vi "Main.vi"() -> ()   [LabVIEW 2020, in "DQMH_API.lvlib"]
uses:
  DQMH_API.lvlib
  Event types--enum.ctl
panel:
  in  "Events":u16(ring) items=["Cloneable Module.lvlib:Do Something.vi", "Cloneable Module.lvlib:Do Something Else.vi", "Cloneable Module.lvlib:Show Panel.vi", "Cloneable Module.lvlib:Hide Panel.vi", "Cloneable Module.lvlib:Stop Module.vi", "Cloneable Module.lvlib:Show Diagram.vi"]
  in  "Event type":T1
  in  "Scan Module Events":bool
  in  "Stop":bool
  in  "Module to work with":u16(ring) items=["Singleton Module.lvlib", "Cloneable Module.lvlib"]
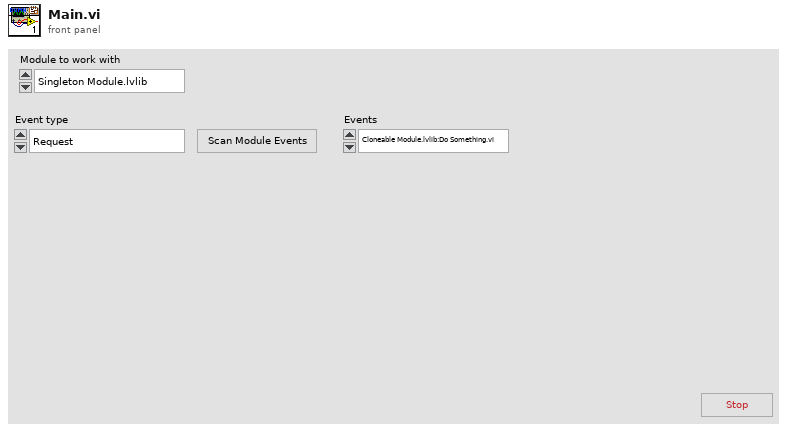
[diagram p1: front panel]
types:
  T1 = typedef "DQMH_API.lvlib/Event types--enum.ctl" = enum16{"Request", "Request and Wait for Reply", "Broadcast"}
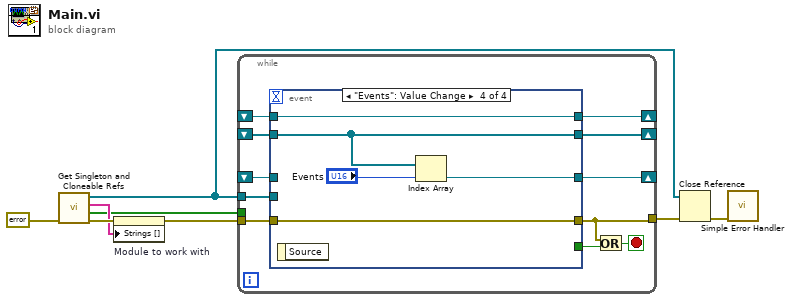
[diagram p0: block diagram]
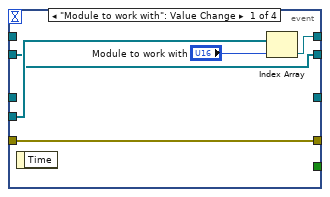
[diagram p2: hidden frame]
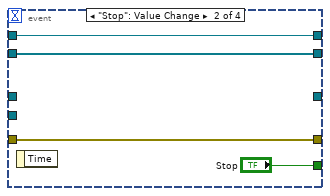
[diagram p3: hidden frame]
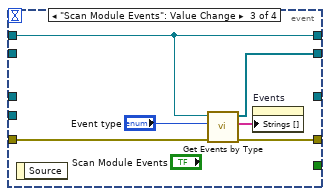
[diagram p4: hidden frame]
diagram:
  n1 = call "Get Singleton and Cloneable Refs.vi"("error in"=errorcluster {"status"=FALSE, "code"=0, "source"=""}) -> ("error out"=w6:errorcluster, "Cloneable?"=w2:bool[], "Modules List"=w3:string[], "DQMH Modules"=w1:refnum<vi>[])  [unwired: 7 in]
  n2 = property on="Module to work with" class="Ring (strict)"(error in=w6, "Strings []"=w3) -> (error out=w7:errorcluster)  [unwired: 1 in, 1 out]
  n3 = while {
    tunnel: w1 -> [w17]
    tunnel: w7 -> [w19]
    tunnel: w2 -> [_]
    tunnel: [w18] -> w5
    shift-right: [w15] -> _
    shift-left: _ -> [w13]
    shift-right: [w12] -> _
    shift-left: _ -> [w11]
    shift-right: [w10] -> _
    shift-left: _ -> [w9]
    stop <- w14 stop-if-true
    n4 = event shown="[3] \"Events\": Value Change" {
      selector: _ -> [_ _ _ _]
      dyn-events: _ -> [_ _ _ _]
      timeout: _ -> [_ _ _ _]
      tunnel: w17 -> [w23 _ _ _]
      tunnel: [_ "Stop" _ _] -> w16
      tunnel: [w21 w26 w31 w37] -> w15
      tunnel: w19 -> [w24 w28 w34 w36]
      tunnel: [w24 w28 w33 w36] -> w18
      tunnel: w13 -> [_ w26 w31 w37]
      tunnel: [w20 w25 w29 w38] -> w12
      tunnel: w11 -> [w20 w25 _ w38]
      tunnel: [_ _ _ w35] -> w10
      tunnel: w9 -> [_ _ _ _]
      event "Module to work with": Value Change {
        n5 = event-data() -> ()  [unwired: 1 in, 1 out]
        n6 = Index Array(array=w23, index="Module to work with") -> (element=w21:refnum<vi>)
      }
      event "Stop": Value Change {
        n7 = event-data() -> ()  [unwired: 1 in, 1 out]
      }
      event "Scan Module Events": Value Change {
        n8 = event-data() -> ()  [unwired: 1 in, 1 out]
        n9 = call "Get Events by Type.vi"("error in"=w34, "Event type"="Event type", "DQMH Module Ref"=w31) -> ("error out"=w33:errorcluster, "Event Name"=w30:string[], "Event Ref"=w29:refnum<vi>[])  [unwired: 6 in]
        n10 = property on="Events" class="Ring (strict)"("Strings []"=w30) -> ()  [unwired: 2 in, 2 out]
      }
      event "Events": Value Change {
        n11 = event-data() -> ()  [unwired: 1 in, 1 out]
        n12 = Index Array(array=w38, index="Events") -> (element=w35:refnum<vi>)
      }
    }
    n13 = Or(x=w18, y=w16) -> (x .or. y?=w14:bool)
  }
  n14 = Close Reference(reference=w1, error in (no error)=w5) -> (error out=w4:errorcluster)
  n15 = call <vilib>:"Simple Error Handler.vi"("error in (no error)"=w4) -> ()  [unwired: 4 in, 5 out]
